vi "Draw Intensity Plot.vi"(7 "Offsets":cluster{"X offset":i16, "Y offset":i16}, 8 "error in":errorcluster, 10 "Data":u32[][](array[numeric]), 11 "picture in":picture) -> (0 "error out":errorcluster, 3 "picture out":picture)   [LabVIEW 2009]
doc: "This VI draws an intensity plot on a picture control. The VI takes an initial picture, a set of offsets into the picture, and 2-D array of colors. The VI returns a picture containing the intensity plot."
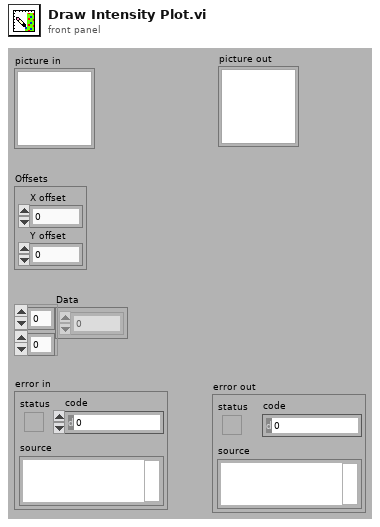
[diagram p1: front panel]
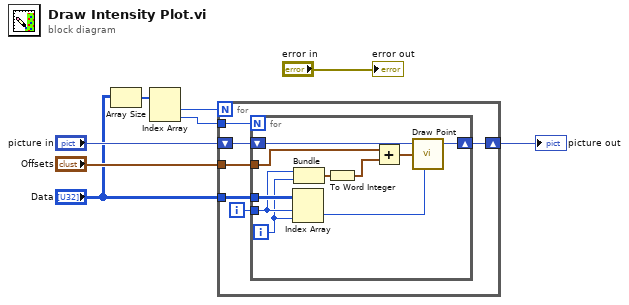
[diagram p0: block diagram]
diagram:
  n1 = Array Size(array="Data") -> (size(s)=w4:i32[])
  n2 = Index Array(array=w4) -> (element #1=w5:i32, element #2=w6:i32)  [unwired: 2 in]
  n3 = for {
    N: w5 -> [_]
    tunnel: "Data" -> [w14]
    shift-right: [w12] -> w2
    shift-left: "picture in" -> [w11]
    tunnel: w6 -> [w10]
    tunnel: "Offsets" -> [w9]
    i -> [w13]
    n4 = for {
      N: w10 -> [_]
      tunnel: w14 -> [w24]
      tunnel: w13 -> [w22]
      shift-right: [w20] -> w12
      shift-left: w11 -> [w19]
      tunnel: w9 -> [w15]
      i -> [w21]
      n5 = Index Array(array=w24, index (row)=w22, index (col)=w21) -> (element=w23:u32)
      n6 = Bundle(w22, w21) -> (w17:cluster{i32, i32})  [unwired: 1 in]
      n7 = To Word Integer(number=w17) -> (16bit integer=w16:cluster{i16, i16})
      n8 = Add(x=w15, y=w16) -> (x+y=w18:cluster{i16, i16})
      n9 = call <vilib>:"Draw Point.vi"("picture"=w19, "point(x,y)"=w18, "color(black)"=w23) -> ("new picture"=w20:picture)  [unwired: 6 in]
    }
  }
  "picture out" <- w2
  "error out" <- "error in"
